vi "FPGA Read Session.vi"(8 "error in (no error)":errorcluster, 11 "FPGA Interface Base in":refnum<class "FPGA Interface Base.lvclass">) -> (0 "error out":errorcluster, 2 "FPGA Session":u32, 3 "FPGA Interface Base out":refnum<class "FPGA Interface Base.lvclass">)   [LabVIEW 2010, in "FPGA Interface Base.lvclass"]
uses:
  <userlib>/_FPGA Interface Advanced Tools/FPGA Interface Base/FPGA Interface Base.lvclass
  <userlib>/_FPGA Interface Advanced Tools/FPGA Interface Base/FPGA Interface Base.lvclass/FPGA Interface Base.ctl
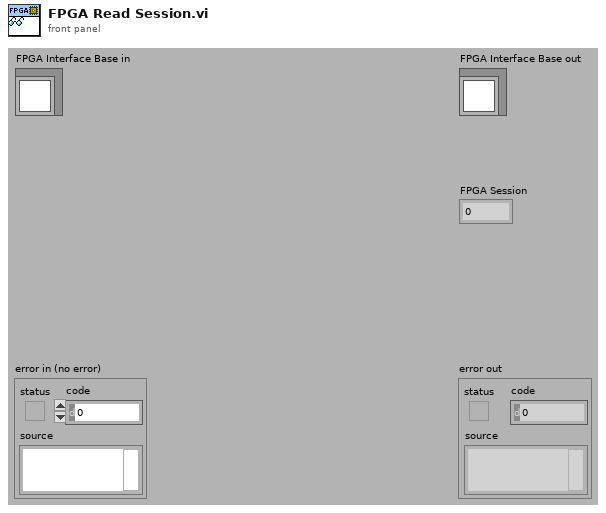
[diagram p1: front panel]
types:
  T1 = typedef "FPGA Interface Base.lvclass/FPGA Session.ctl" = refnum<data-value>
  T2 = typedef "FPGA Interface Base.lvclass/FPGA Session Data.ctl" = cluster{"Session Out":u32, "Indicator Scalars":T3, "Indicator Arrays":T5, "Control Scalars":T3, "Control Arrays":T5, "TargetToHost FIFO Channels":T7, "HostToTarget FIFO Channels":T7, "All FIFOs":T8[], "IRQ Context Queue":refnum<queue>}
  T3 = typedef "FPGA Bitfile Utility.lvlib/Scalar Register Set.ctl" = cluster{"Boolean":T4[], "I8":T4[], "I16":T4[], "I32":T4[], "I64":T4[], "U8":T4[], "U16":T4[], "U32":T4[], "U64":T4[]}
  T4 = typedef "FPGA Bitfile Utility.lvlib/Scalar Register.ctl" = cluster{"Address":u32, "Name":string}
  T5 = typedef "FPGA Bitfile Utility.lvlib/Array Register Set.ctl" = cluster{"Boolean":T6[], "I8":T6[], "I16":T6[], "I32":T6[], "I64":T6[], "U8":T6[], "U16":T6[], "U32":T6[], "U64":T6[]}
  T6 = typedef "FPGA Bitfile Utility.lvlib/Array Register.ctl" = cluster{"Address":u32, "Num Elements":u32, "Name":string}
  T7 = typedef "FPGA Bitfile Utility.lvlib/FIFO Channel Set.ctl" = cluster{"Boolean":T8[], "I8":T8[], "I16":T8[], "I32":T8[], "I64":T8[], "U8":T8[], "U16":T8[], "U32":T8[], "U64":T8[]}
  T8 = typedef "FPGA Bitfile Utility.lvlib/FIFO Channel.ctl" = cluster{"Physical Channel":u32, "Name":string}
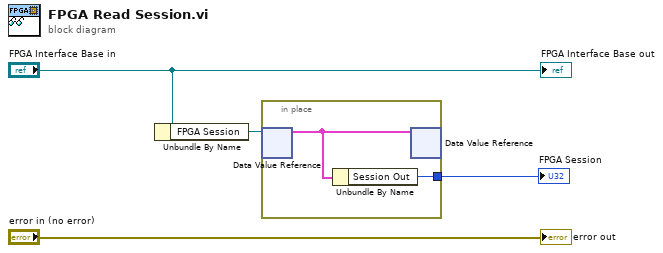
[diagram p0: block diagram]
diagram:
  n1 = Unbundle By Name("FPGA Interface Base in") -> ("FPGA Session"=w2:T1)
  n2 = in-place {
    in-place-border: [w5] -> w3
    n3 = in-place-dvr #1(w2) -> (w6:T2)  [unwired: 1 out]
    n4 = Unbundle By Name(w6) -> ("Session Out"=w5:u32)
    n5 = in-place-dvr #1(w6) -> ()  [unwired: 2 out]
  }
  "FPGA Session" <- w3
  "error out" <- "error in (no error)"
  "FPGA Interface Base out" <- "FPGA Interface Base in"
